vi "Record Frame Crop.vi"(8 "error in (no error)":errorcluster, 10 "Starting frame number":u32, 11 "Frame Grabber Data In in":T1={"Camera Session"="", "Frame"=refnum, "AVI Refnum"=refnum, "Codecs"=[], "Frame number"=0, "Tracking File Refnum"=refnum, "Tick Count"=0, "Probe Object"=refnum, "Playback Probe Data"=[], "Rigid Body"={"Position"={"x (mm)"=0.0, "y (mm)"=0.0, "z (mm)"=0.0}, "Orientation"={"Pitch (rad)"=0.0, "Yaw (rad)"=0.0, "Roll (rad)"=0.0}, "Quaternion"={"qx"=0.0, "qy"=0.0, "qz"=0.0, "qw"=0.0}, "Tracked?"=FALSE}, "Total no frames playback"=0, "Video FPS"=0.0, "Camera connected?"=FALSE, "Scene"=refnum, "Cropped Frame"=refnum, "Tracker FPS"=0.0, "Crop ROI"=[], "Presentation Values"=[], "Elapsed time (ms)"=0, "Camera frames playback"=0, "Refnums"={"Live Refnum"=refnum, "Record Refnum"=refnum, "Playback Refnum"=refnum, "Frame Slider Refnum"=refnum, "Pause Refnum"=refnum, "Home Refnum"=refnum, "Crop Refnum"=refnum, "Clear Crop Refnum"=refnum, "stop refnum"=refnum, "Playback Rate Refnum"=refnum, "Presentation Refnum"=refnum, "Crop Time Frame Slider Refnum"=refnum, "Cancel Save Refnum"=refnum, "Reverse Playback Refnum"=refnum, "Recording Settings Refnum"=refnum}, "Dimensions"={"Probe Dimensions"={"Probe Width"=0.0, "Probe Depth"=1.0, "Probe Height"=0.0}, "Room Dimensions"={"Room Width"=0.0, "Room Depth"=0.0, "Room Height"=0.0}}, "Playback Data As Strings"=[], "Cropped Tracking File Refnum"=refnum, "Cropped AVI Refnum"=refnum, "Header"=[], "Total euclidian distance"=0.0, "Annotation File Path"=path "", "Playback File Path"=path "", "Size per frame"=0.0}) -> (0 "error out":errorcluster, 2 "Cancel save?":bool, 3 "Frame Grabber Data out":T1={"Camera Session"="", "Frame"=refnum, "AVI Refnum"=refnum, "Codecs"=[], "Frame number"=0, "Tracking File Refnum"=refnum, "Tick Count"=0, "Probe Object"=refnum, "Playback Probe Data"=[], "Rigid Body"={"Position"={"x (mm)"=0.0, "y (mm)"=0.0, "z (mm)"=0.0}, "Orientation"={"Pitch (rad)"=0.0, "Yaw (rad)"=0.0, "Roll (rad)"=0.0}, "Quaternion"={"qx"=0.0, "qy"=0.0, "qz"=0.0, "qw"=0.0}, "Tracked?"=FALSE}, "Total no frames playback"=0, "Video FPS"=0.0, "Camera connected?"=FALSE, "Scene"=refnum, "Cropped Frame"=refnum, "Tracker FPS"=0.0, "Crop ROI"=[], "Presentation Values"=[], "Elapsed time (ms)"=0, "Camera frames playback"=0, "Refnums"={"Live Refnum"=refnum, "Record Refnum"=refnum, "Playback Refnum"=refnum, "Frame Slider Refnum"=refnum, "Pause Refnum"=refnum, "Home Refnum"=refnum, "Crop Refnum"=refnum, "Clear Crop Refnum"=refnum, "stop refnum"=refnum, "Playback Rate Refnum"=refnum, "Presentation Refnum"=refnum, "Crop Time Frame Slider Refnum"=refnum, "Cancel Save Refnum"=refnum, "Reverse Playback Refnum"=refnum, "Recording Settings Refnum"=refnum}, "Dimensions"={"Probe Dimensions"={"Probe Width"=0.0, "Probe Depth"=1.0, "Probe Height"=0.0}, "Room Dimensions"={"Room Width"=0.0, "Room Depth"=0.0, "Room Height"=0.0}}, "Playback Data As Strings"=[], "Cropped Tracking File Refnum"=refnum, "Cropped AVI Refnum"=refnum, "Header"=[], "Total euclidian distance"=0.0, "Annotation File Path"=path "", "Playback File Path"=path "", "Size per frame"=0.0})   [LabVIEW 2017]
uses:
  Controls/Frame Grabber Data.ctl
  <vilib>/userdefined/High Color/IMAQdx.ctl
  <vilib>/vision/Image Controls.llb/IMAQ Image.ctl
  <vilib>/vision/Avi.llb/IMAQ AVI2 Refnum.ctl
  Controls/Rigid Body Info.ctl
  Controls/Position.ctl
  Controls/Orientation.ctl
  Controls/Refnums.ctl
  Controls/Recording Settings.ctl
  Controls/Operator Settings.ctl
  Controls/Operator.ctl
  Controls/Patient Settings.ctl
  Controls/Dimensions.ctl
  Controls/Room Dimensions.ctl
  <vilib>/vision/NI_Vision_Development_Module.lvlib
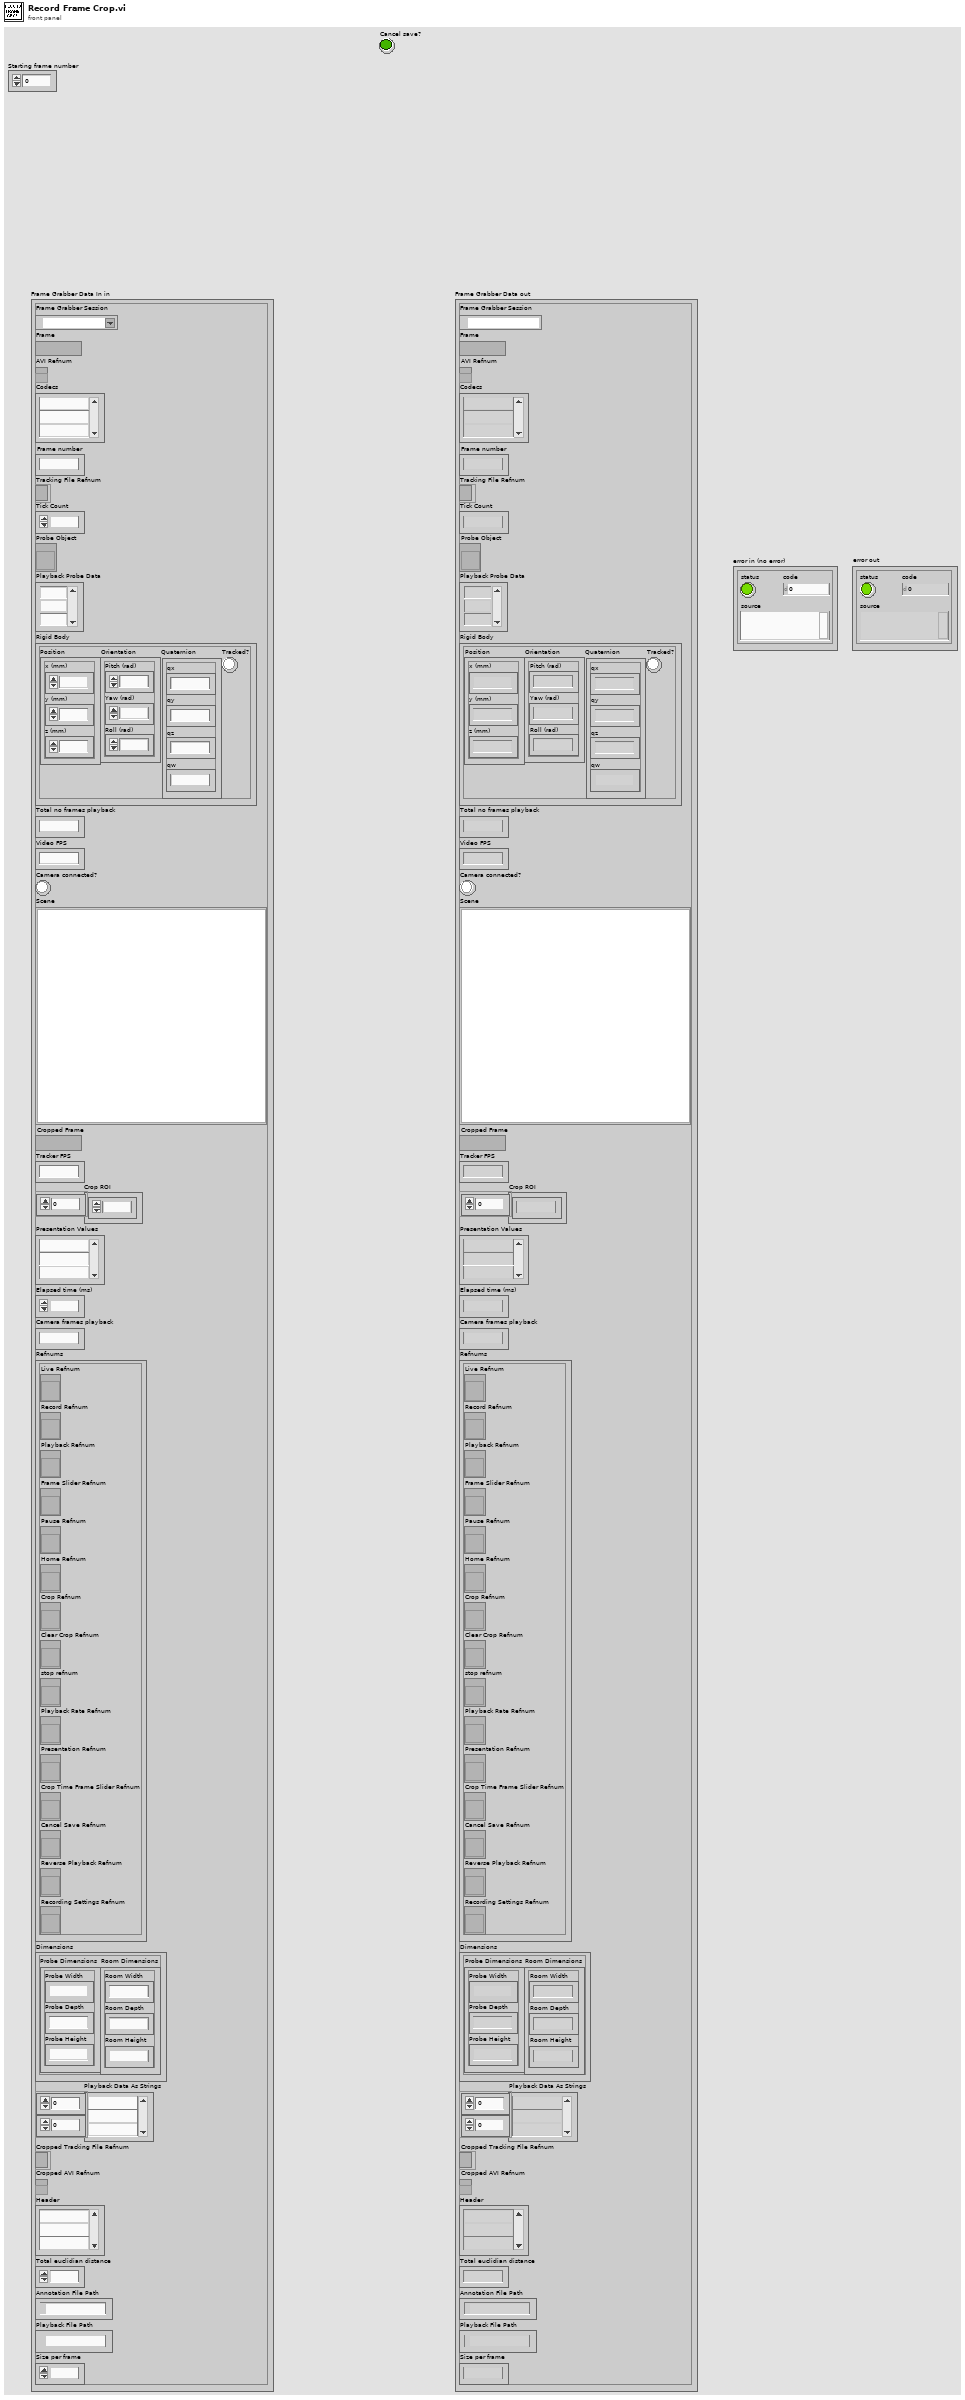
[diagram p1: front panel]
types:
  T1 = typedef "Frame Grabber Data.ctl" = cluster{"Camera Session":T2, "Frame":T3, "AVI Refnum":T4, "Codecs":string[], "Frame number":u32, "Tracking File Refnum":refnum<file>, "Tick Count":u32, "Probe Object":refnum<vi>, "Playback Probe Data":dbl[][], "Rigid Body":T5, "Total no frames playback":i32, "Video FPS":dbl, "Camera connected?":bool, "Scene":refnum<vi>, "Cropped Frame":T3, "Tracker FPS":dbl, "Crop ROI":i32[], "Presentation Values":string[], "Elapsed time (ms)":u32, "Camera frames playback":u32, "Refnums":T8, "Dimensions":T9, "Playback Data As Strings":string[][], "Cropped Tracking File Refnum":refnum<file>, "Cropped AVI Refnum":T4, "Header":string[], "Total euclidian distance":dbl, "Annotation File Path":path, "Playback File Path":path, "Size per frame":dbl}
  T2 = typedef "IMAQdx.ctl" = refnum<k21>
  T3 = typedef "IMAQ Image.ctl" = refnum<image>
  T4 = typedef "IMAQ AVI2 Refnum.ctl" = refnum<k20>
  T5 = typedef "Rigid Body Info.ctl" = cluster{"Position":T6, "Orientation":T7, "Quaternion":cluster{"qx":sgl, "qy":sgl, "qz":sgl, "qw":sgl}, "Tracked?":bool}
  T6 = typedef "Position.ctl" = cluster{"x (mm)":sgl, "y (mm)":sgl, "z (mm)":sgl}
  T7 = typedef "Orientation.ctl" = cluster{"Pitch (rad)":sgl, "Yaw (rad)":sgl, "Roll (rad)":sgl}
  T8 = typedef "Refnums.ctl" = cluster{"Live Refnum":refnum<vi>, "Record Refnum":refnum<vi>, "Playback Refnum":refnum<vi>, "Frame Slider Refnum":refnum<vi>, "Pause Refnum":refnum<vi>, "Home Refnum":refnum<vi>, "Crop Refnum":refnum<vi>, "Clear Crop Refnum":refnum<vi>, "stop refnum":refnum<vi>, "Playback Rate Refnum":refnum<vi>, "Presentation Refnum":refnum<vi>, "Crop Time Frame Slider Refnum":refnum<vi>, "Cancel Save Refnum":refnum<vi>, "Reverse Playback Refnum":refnum<vi>, "Recording Settings Refnum":refnum<vi>}
  T9 = typedef "Dimensions.ctl" = cluster{"Probe Dimensions":cluster{"Probe Width":sgl, "Probe Depth":sgl, "Probe Height":sgl}, "Room Dimensions":T10}
  T10 = typedef "Room Dimensions.ctl" = cluster{"Room Width":dbl, "Room Depth":dbl, "Room Height":dbl}
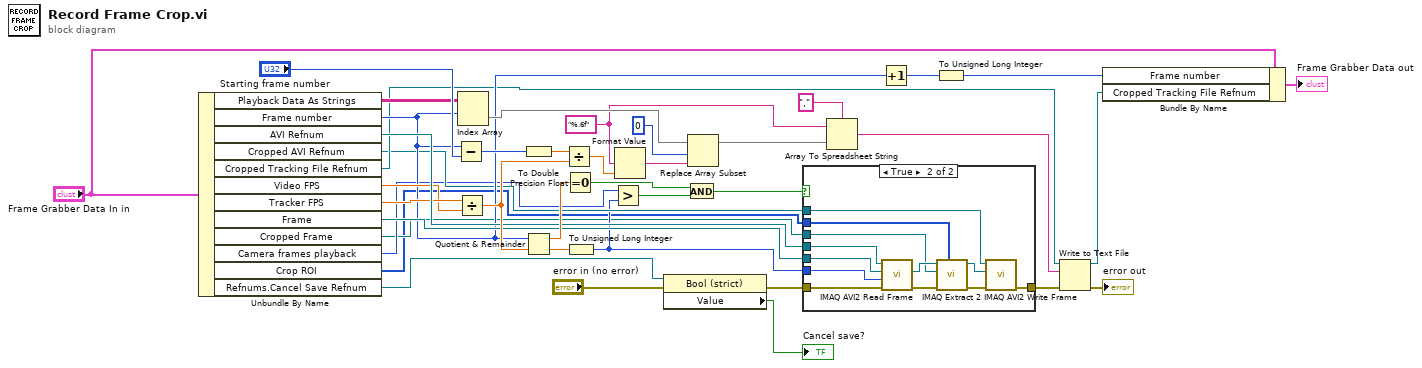
[diagram p0: block diagram]
diagram:
  w11 = "%.6f" ("format string")
  n1 = Unbundle By Name("Frame Grabber Data In in") -> ("Playback Data As Strings"=w24:string[][], "Frame number"=w18:u32, "AVI Refnum"=w29:T4, "Cropped AVI Refnum"=w12:T4, "Cropped Tracking File Refnum"=w13:refnum<file>, "Video FPS"=w26:dbl, "Tracker FPS"=w27:dbl, "Frame"=w30:T3, "Cropped Frame"=w6:T3, "Camera frames playback"=w8:u32, "Crop ROI"=w5:i32[], "Refnums.Cancel Save Refnum"=w3:refnum<vi>)
  n2 = Subtract(x=w18, y="Starting frame number") -> (x-y=w19:u32)
  n3 = Divide(x=w27, y=w26) -> (x/y=w35:dbl)
  n4 = Index Array(array=w24, index (row)=w18) -> (element=w23:string[])  [unwired: 1 in]
  n5 = To Double Precision Float(number=w19) -> (double precision float=w34:dbl)
  n6 = Quotient & Remainder(x=w18, y=w35) -> (x-y*floor(x/y)=w36:dbl, floor(x/y)=w31:dbl)
  n7 = Divide(x=w34, y=w35) -> (x/y=w33:dbl)
  n8 = Equal To 0?(x=w36) -> (x = 0?=w32:bool)
  n9 = To Unsigned Long Integer(number=w31) -> (unsigned 32bit integer=w9:u32)
  n10 = Greater?(x=w8, y=w9) -> (0:w7:bool)
  n11 = Format Value(format string=w11, value (0)=w33) -> (output string=w21:string)  [unwired: 1 in]
  n12 = property class="Bool (strict)"(reference=w3, error in="error in (no error)") -> (error out=w2:errorcluster, "Value"=→"Cancel save?":bool)  [unwired: 1 out]
  n13 = And(x=w32, y=w7) -> (x .and. y?=w10:bool)
  n14 = Replace Array Subset(array=w23, new element=w21, index=0) -> (w16:string[])
  n15 = case shown="True" w10 {
    tunnel: [w41 w53] -> w40
    tunnel: w2 -> [w41 w52]
    tunnel: w30 -> [_ w51]
    tunnel: w29 -> [_ w50]
    tunnel: w9 -> [_ w49]
    tunnel: w12 -> [_ w48]
    tunnel: w6 -> [_ w43]
    tunnel: w5 -> [_ w42]
    frame False {
    }
    frame True {
      n16 = call "IMAQ AVI2 Read Frame"("error in (no error)"=w52, "Frame Number"=w49, "Image"=w51, "AVI Refnum"=w50) -> ("error out"=w47:errorcluster, "Image Out"=w45:T3)  [unwired: 5 in, 1 out]
      n17 = call "IMAQ Extract 2"("Optional Rectangle"=w42, "error in (no error)"=w47, "Image Dst"=w43, "Image Src"=w45) -> ("error out"=w46:errorcluster, "Image Dst Out"=w44:T3)  [unwired: 6 in]
      n18 = call "IMAQ AVI2 Write Frame"("error in (no error)"=w46, "Image"=w44, "AVI Refnum"=w48) -> ("error out"=w53:errorcluster)  [unwired: 6 in, 2 out]
    }
  }
  n19 = Array To Spreadsheet String(delimiter (Tab)=",", array=w16, 3:w11) -> (spreadsheet string=w14:string)
  n20 = Increment(x=w18) -> (x+1=w37:u32)
  n21 = To Unsigned Long Integer(number=w37) -> (unsigned 32bit integer=w20:u32)
  n22 = Write to Text File(file (use dialog)=w13, text=w14, error in=w40) -> (refnum out=w39:refnum<file>, error out=→"error out":errorcluster)  [unwired: 1 in, 1 out]
  n23 = Bundle By Name(cluster="Frame Grabber Data In in", "Frame number"=w20, "Cropped Tracking File Refnum"=w39) -> (→"Frame Grabber Data out":T1)
